vi "Actor Core.vi"(8 "error in":errorcluster, 11 "Nested in":refnum<class "CheckPasswordUI.lvclass">) -> (0 "error out":errorcluster, 3 "Actor out":refnum<class "Actor.lvclass">)   [LabVIEW 2021, in "CheckPasswordUI.lvclass"]
doc: "(<B>Filename</B>: Actor Framework.lvlib:Actor.lvclass:Actor Core.vi)\n\nReceives messages to the actor, reacts to them, and initiates any error handling that may shut the actor down.\n\nDescendant classes may override this VI to append parallel tasks for the actor to complete while it handles messages. Overrides use the Call Parent Method node."
uses:
  CheckPasswordUI.lvclass
  C:/Program Files (x86)/National Instruments/LabVIEW 2021/user.lib/John_Lib/AbstractActorTemplate/AbstractActorTemplate/UIActorTop.lvclass
  C:/Program Files (x86)/National Instruments/LabVIEW 2021/vi.lib/ActorFramework/Actor/Actor.lvclass
  <vilib>/ActorFramework/Actor/Actor.lvclass
  CheckUser.ctl
  TopRef.ctl
  CheckPasswordUI.lvclass/CheckPasswordUI.ctl
  <vilib>/ActorFramework/Actor/Actor.lvclass/Actor.ctl
  <vilib>/ActorFramework/Message Enqueuer/Message Enqueuer.lvclass/Message Enqueuer.ctl
  <vilib>/ActorFramework/Message Enqueuer/Init from Existing Queue.vi
  <vilib>/ActorFramework/Message Enqueuer/Enqueue.vi
  <vilib>/ActorFramework/Stop Msg/Stop Msg.lvclass
  C:/Program Files (x86)/National Instruments/LabVIEW 2021/vi.lib/ActorFramework/Message/Message.lvclass
  <vilib>/Utility/LVClass/Get LV Class Name.vi
  <resource>/AFDebug/Generate Trace for Message.vi
  <vilib>/ActorFramework/Message Priority Queue/Priority Enqueue.vi
  <userlib>/John_Lib/Queue_Self/Q-StringToArray_Sushu.vi
  <vilib>/ActorFramework/Message Enqueuer/Message Enqueuer.lvclass
  <userlib>/John_Lib/AbstractActorTemplate/AbstractActorTemplate/UIActorTop.lvclass
  <userlib>/John_Lib/Queue_Self/Queue_Self.lvlib
panel:
  in  "CheckUser":T1
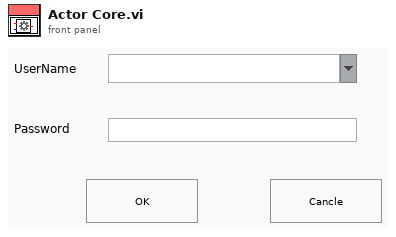
[diagram p1: front panel]
types:
  T1 = typedef "CheckPasswordUI.lvclass/CheckUser.ctl" = cluster{"UserName":string, "Password":string, "OK":bool, "Cancle":bool, "Messages":string}
  T2 = typedef "CheckPasswordUI.lvclass/TopRef.ctl" = cluster{"CheckUser":refnum<vi>, "Str Messages":refnum<vi>, "Str Password":refnum<vi>}
  T3 = typedef "LVRectTypeDef.ctl" = cluster{"Left":i16, "Top":i16, "Right":i16, "Bottom":i16}
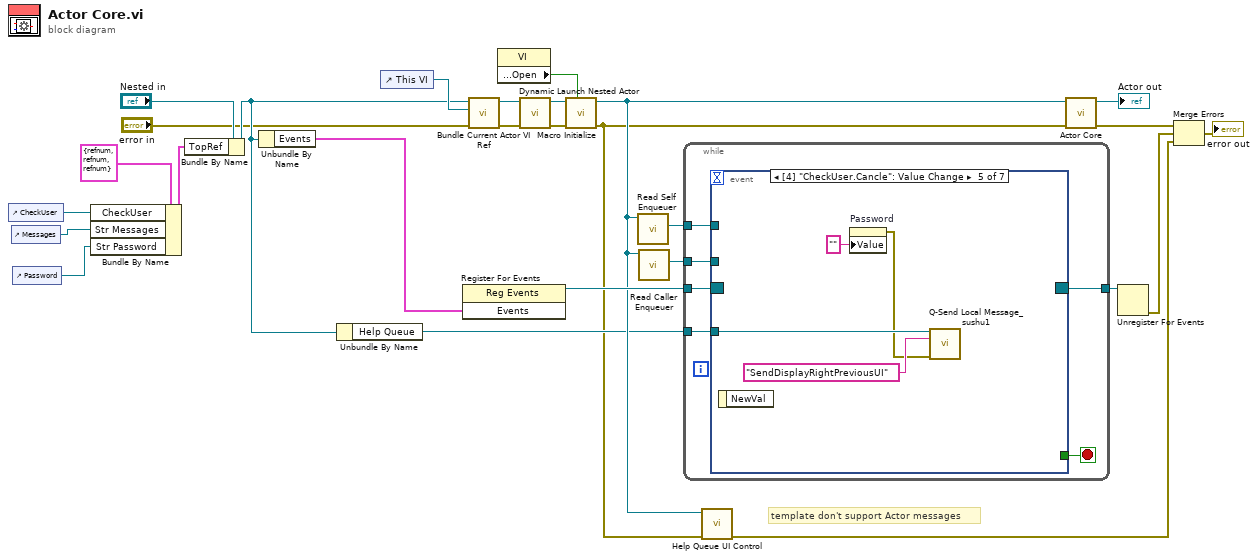
[diagram p0: block diagram]
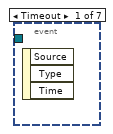
[diagram p2: hidden frame]
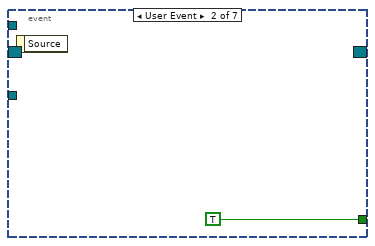
[diagram p3: hidden frame]
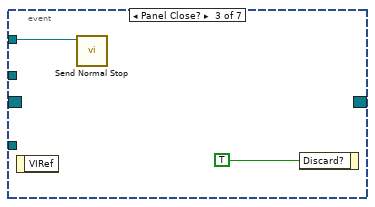
[diagram p4: hidden frame]
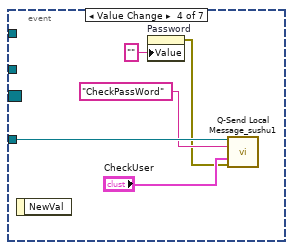
[diagram p5: hidden frame]
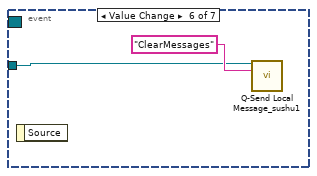
[diagram p6: hidden frame]
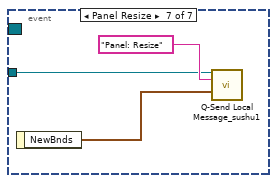
[diagram p7: hidden frame]
diagram:
  # "template don't support Actor messages"
  n1 = control-ref of="CheckUser"() -> (w9:refnum<vi>)
  n2 = control-ref of="Messages"() -> (w3:refnum<vi>)
  n3 = control-ref of="Password"() -> (w2:refnum<vi>)
  n4 = Bundle By Name(cluster=T2 {"CheckUser"=refnum, "Str Messages"=refnum, "Str Password"=refnum} ("TopRef"), "CheckUser"=w9, "Str Messages"=w3, "Str Password"=w2) -> (w10:T2)
  n5 = Bundle By Name(cluster="Nested in", "TopRef"=w10) -> (w6:refnum<class "CheckPasswordUI.lvclass">)
  n6 = Unbundle By Name(w6) -> ("Events"=w25:cluster{"Stop":refnum<user-event>})
  n7 = Unbundle By Name(w6) -> ("Help Queue"=w5:refnum<queue>)
  n8 = control-ref of="This VI"() -> (w12:refnum<vi>)
  n9 = register-events ("Main Register for Events")(w25) -> (reference out=w26:refnum<event-registration>)  [unwired: 2 in, 1 out]
  n10 = call <userlib>:"Bundle Current Actor VI Ref.vi"("error in (no error)"="error in", "This VI"=w12, "UI ActorTop in"=w6) -> ("error out"=w13:errorcluster, "UI ActorTop out"=w14:refnum<class "CheckPasswordUI.lvclass">)  [unwired: 5 in, 2 out]
  n11 = property class="VI"() -> ("Front Panel.Open"=w20:bool)  [unwired: 2 in, 2 out]
  n12 = call-dynamic "Dynamic Launch Nested Actor.vi"("error in (no error)"=w13, "UI ActorTop in"=w14) -> ("error out"=w21:errorcluster, "UI ActorTop out"=w22:refnum<class "CheckPasswordUI.lvclass">)  [unwired: 8 in]
  n13 = call-dynamic "Macro Initialize.vi"("Front Panel Window:Open"=w20, "error in (no error)"=w21, "UI ActorTop in"=w22) -> ("error out"=w4:errorcluster, "UI ActorTop out"=w7:refnum<class "CheckPasswordUI.lvclass">)  [unwired: 7 in]
  n14 = call <vilib>:"Read Self Enqueuer.vi"("Actor"=w7) -> ("Self Enqueuer"=w23:refnum<class "Message Enqueuer.lvclass">)  [unwired: 10 in]
  n15 = call <vilib>:"Read Caller Enqueuer.vi"("Actor"=w7) -> ("Caller Enqueuer"=w16:refnum<class "Message Enqueuer.lvclass">)  [unwired: 10 in]
  n16 = while {
    tunnel: w26 -> [w33]
    tunnel: [w31] -> w24
    tunnel: w23 -> [w30]
    tunnel: w16 -> [w29]
    tunnel: w5 -> [w28]
    stop <- w32 stop-if-true
    n17 = event "UI Events" shown="[4] \"CheckUser.Cancle\": Value Change" {
      selector: w33 -> [_ _ _ _ _ _ _]
      dyn-events: [_ _ _ _ _ _ _] -> w31
      timeout: _ -> [_ _ _ _ _ _ _]
      tunnel: [_ TRUE _ _ _ _ _] -> w32
      tunnel: w30 -> [_ _ w35 _ _ _ _]
      tunnel: w29 -> [_ _ _ _ _ _ _]
      tunnel: w28 -> [_ _ _ w41 w45 w46 w48]
      event Timeout {
        n18 = event-data() -> ()  [unwired: 1 in, 3 out]
      }
      event User Event {
        n19 = event-data() -> ()  [unwired: 1 in, 1 out]
      }
      event Panel Close? {
        n20 = event-data() -> ()  [unwired: 1 in, 1 out]
        n21 = call <vilib>:"Send Normal Stop.vi"("Message Enqueuer"=w35) -> ()  [unwired: 10 in, 1 out]
        n22 = event-data("Discard?"=TRUE) -> ()  [unwired: 1 in, 1 out]
      }
      event Value Change {
        n23 = event-data() -> ()  [unwired: 1 in, 1 out]
        n24 = property on="Password" class="Str"("Value"="") -> (error out=w37:errorcluster)  [unwired: 2 in, 1 out]
        n25 = call <userlib>:"Q-Send Local Message_sushu1.vi"("queue in"=w41, "Elements at Back"="CheckPassWord", "message value"="CheckUser", "error in"=w37) -> ()  [unwired: 9 in, 3 out]
      }
      event Value Change {
        n26 = event-data() -> ()  [unwired: 1 in, 1 out]
        n27 = property on="Password" class="Str"("Value"="") -> (error out=w42:errorcluster)  [unwired: 2 in, 1 out]
        n28 = call <userlib>:"Q-Send Local Message_sushu1.vi"("queue in"=w45, "Elements at Back"="SendDisplayRightPreviousUI", "error in"=w42) -> ()  [unwired: 10 in, 3 out]
      }
      event Value Change {
        n29 = event-data() -> ()  [unwired: 1 in, 1 out]
        n30 = call <userlib>:"Q-Send Local Message_sushu1.vi"("queue in"=w46, "Elements at Back"="ClearMessages") -> ()  [unwired: 11 in, 3 out]
      }
      event Panel Resize {
        n31 = event-data() -> ("NewBnds"=w50:T3)  [unwired: 1 in]
        n32 = call <userlib>:"Q-Send Local Message_sushu1.vi"("queue in"=w48, "Elements at Back"="Panel: Resize", "message value"=w50) -> ()  [unwired: 10 in, 3 out]
      }
    }
  }
  n33 = call "Help Queue UI Control.vi"("error In"=w4, "CheckPasswordUI.lvclass"=w7) -> ("error out"=w8:errorcluster)  [unwired: 9 in]
  n34 = call-parent "Actor Core.vi"("error in"=w4, "Actor in"=w7) -> ("error out"=w18:errorcluster, "Actor out"=→"Actor out":refnum<class "Actor.lvclass">)  [unwired: 8 in]
  n35 = Unregister For Events(event registration refnum=w24) -> (error out=w19:errorcluster)  [unwired: 1 in]
  n36 = Merge Errors(w18, w19, w8) -> (→"error out":errorcluster)
